vi "Example Play File.vi"() -> ()   [LabVIEW 2014]
uses:
  <vilib>/LabVIEW Universal Transcriptor/LabVIEW to Arduino Transcriptor/Transcriptors/System API/Serial println string.vi
  TMRpcm.lvlib
  <vilib>/LabVIEW Universal Transcriptor/LabVIEW Universal Transcriptor SD Card Library/LabVIEW Universal Transcriptor SD Card Library.lvlib
panel:
  out "Error Out":errorcluster
  in  "filename":string="1.wav"
  in  "Error In":errorcluster
  # "max 8 characters together with file extension"
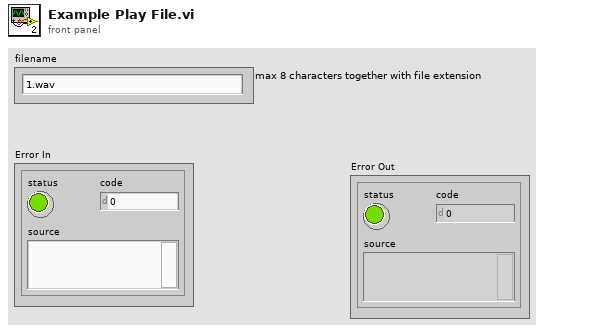
[diagram p1: front panel]
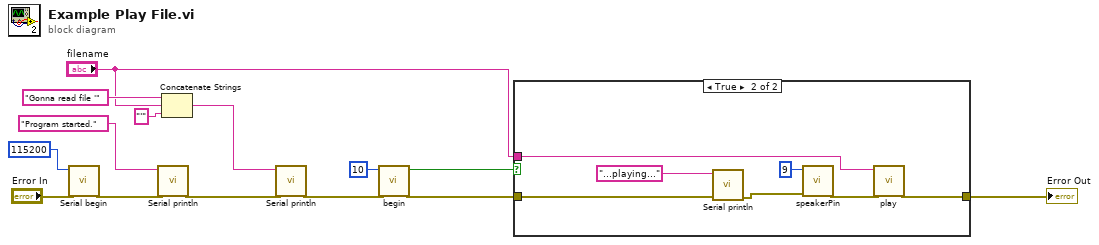
[diagram p0: block diagram]
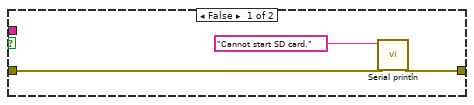
[diagram p2: hidden frame]
diagram:
  n1 = call <vilib>:"Serial begin.vi"("Error In"="Error In", "speed (Bd)"=115200) -> ("Error Out"=w12:errorcluster)  [unwired: 9 in]
  n2 = call-poly <vilib>:"Serial println.vi"("Error In"=w12, "string in"="Program started.") -> ("Error Out"=w8:errorcluster)  [unwired: 9 in]
  n3 = Concatenate Strings("Gonna read file '" ("string"), "filename", "'" ("string")) -> (w5:string)
  n4 = call-poly <vilib>:"Serial println.vi"("Error In"=w8, "string in"=w5) -> ("Error Out"=w2:errorcluster)  [unwired: 9 in]
  n5 = call <vilib>:"begin.vi"("Error In"=w2, "CS pin (optional)"=u8 10) -> ("Error Out"=w3:errorcluster, "success?"=w1:bool)  [unwired: 8 in]
  n6 = case shown="True" w1 {
    tunnel: [w16 w24] -> w14
    tunnel: "filename" -> [_ w23]
    tunnel: w3 -> [w17 w19]
    frame False {
      n7 = call-poly <vilib>:"Serial println.vi"("Error In"=w17, "string in"="Cannot start SD card.") -> ("Error Out"=w16:errorcluster)  [unwired: 9 in]
    }
    frame True {
      n8 = call-poly <vilib>:"Serial println.vi"("Error In"=w19, "string in"="...playing...") -> ("Error Out"=w18:errorcluster)  [unwired: 9 in]
      n9 = call "speakerPin.vi"("Error In"=w18, "speakerPin"=u8 9) -> ("Error Out"=w22:errorcluster)  [unwired: 9 in]
      n10 = call "play.vi"("Error In"=w22, "filename"=w23) -> ("Error Out"=w24:errorcluster)  [unwired: 9 in]
    }
  }
  "Error Out" <- w14
